vi "Configure Average.vi"(7 "Average on":bool, 8 "error in (no error)":errorcluster, 10 "Average Count":i32, 11 "Power Meter in":refnum<class "Power Meter.lvclass">) -> (0 "error out":errorcluster, 3 "Power Meter out":refnum<class "Power Meter.lvclass">)   [LabVIEW 2020, in "Power Meter.lvclass"]
uses:
  Power Meter.lvclass
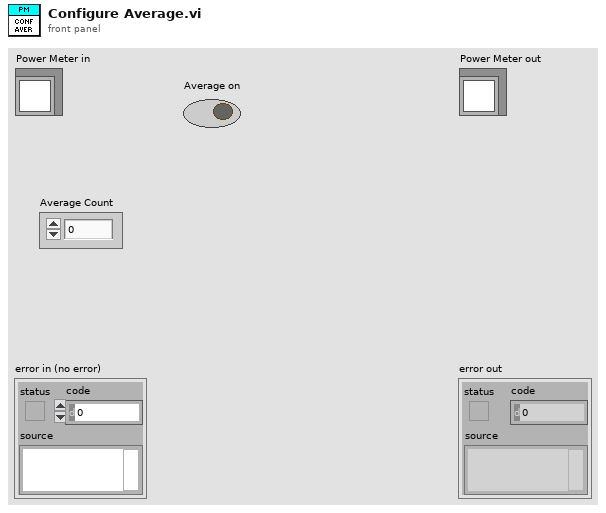
[diagram p1: front panel]
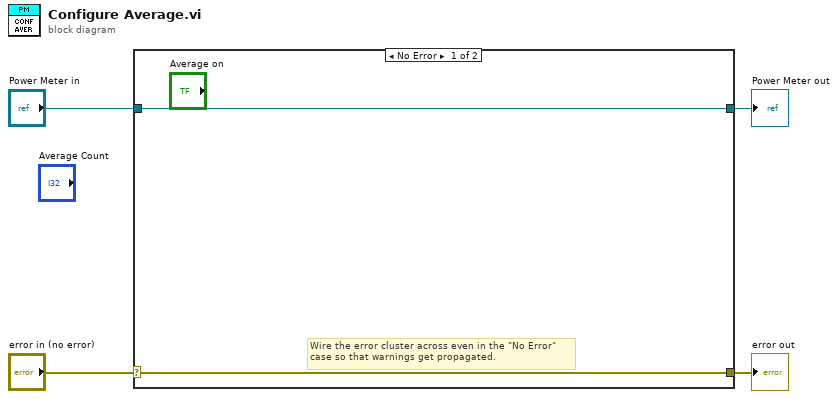
[diagram p0: block diagram]
diagram:
  n1 = case shown="No Error" "error in (no error)" {
    selector: "error in (no error)" -> [w5 w8]
    tunnel: [w5 w8] -> w3
    tunnel: [w6 w7] -> w1
    tunnel: "Power Meter in" -> [w6 w7]
    frame No Error {
      # "Wire the error cluster across even in the \"No Error\"\ncase so that warnings get propagated."
    }
    frame Error {
    }
  }
  "error out" <- w3
  "Power Meter out" <- w1
